vi "ABCtoAlphaBeta_3PhasePowerInvariant_src.vi"(0 "A":sgl, 5 "B":sgl, 7 "C":sgl) -> (4 "alpha":sgl, 6 "beta":sgl)   [LabVIEW 2017]
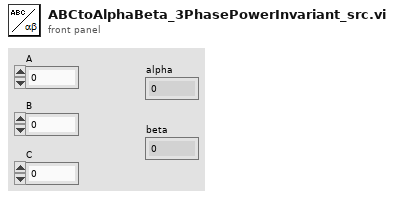
[diagram p1: front panel]
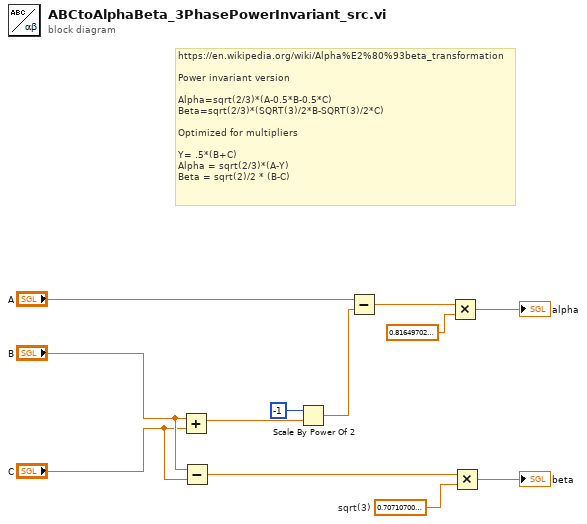
[diagram p0: block diagram]
diagram:
  w8 = sgl 0.707107  # sqrt(3)
  # "https://en.wikipedia.org/wiki/Alpha%E2%80%93beta_transformation\n\nPower invariant version\n\nAlpha=sqrt(2/3)*(A-0.5*B-0.5*C)\nBeta=sqrt(2/3)*(SQRT(3)/2*B-SQRT(3)/2*C)\n\nOptimized for multipliers\n\nY= .5*(B+C)\nAlpha = sqrt(2/3)*(A-Y)\nBeta = sqrt(2)/2 * (B-C)"
  n1 = Add(x="B", y="C") -> (x+y=w6:sgl)
  n2 = Subtract(x="B", y="C") -> (x-y=w7:sgl)
  n3 = Scale By Power Of 2(n=i16 -1, x=w6) -> (x*2^n=w4:sgl)
  n4 = Subtract(x="A", y=w4) -> (x-y=w2:sgl)
  n5 = Multiply(x=w2, y=sgl 0.816497) -> (x*y=→"alpha":sgl)
  n6 = Multiply(x=w7, y=w8) -> (x*y=→"beta":sgl)
